vi "setReset.vi"(8 "error":errorcluster, 10 "axis":i32, 11 "connection ID":refnum<k5>) -> (0 "error out":errorcluster, 2 "axis_out":i32, 3 "connection ID out":refnum<k5>)   [LabVIEW 2016, in "amc_api.lvlib"]
doc: "This function resets the actual position of the selected axis given by the NUM sensor to zero and marks the reference position as invalid."
uses:
  amc_api.lvlib
panel:
  out "jsonRespIn":string
  out "JSON-response":string="{\"jsonrpc\":\"2.0\",\"method\":\"\",\"params\":[5,1.245,true,\"name\"],\"id\":\"1\"}"
  out "JSON request":string
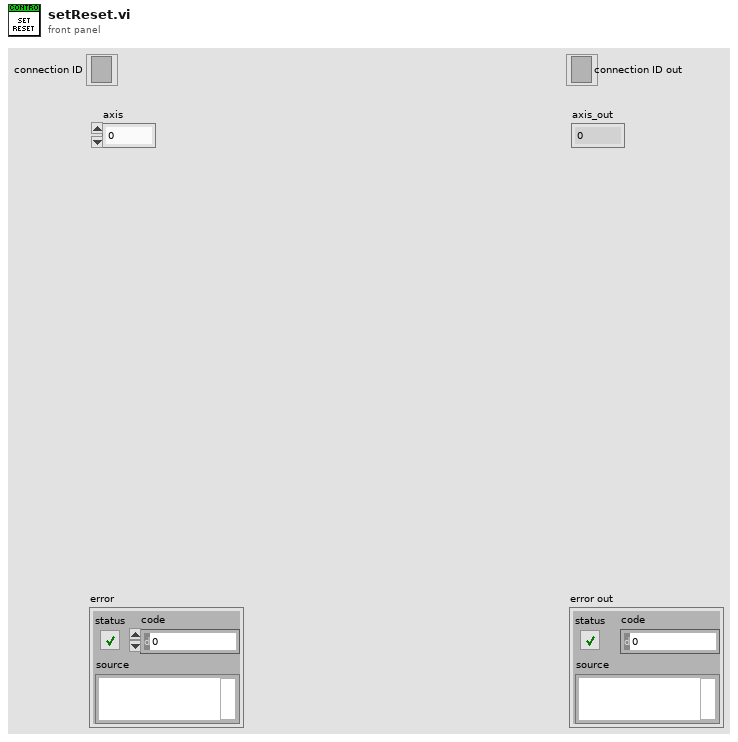
[diagram p1: front panel]
types:
  T1 = cluster{"jsonrpc":string, "method":string, "params":string[], "id":string, "api":i32, "pid":string}
  T2 = enum16{"Standard", "Buffered", "CRLF", "Immediate"}
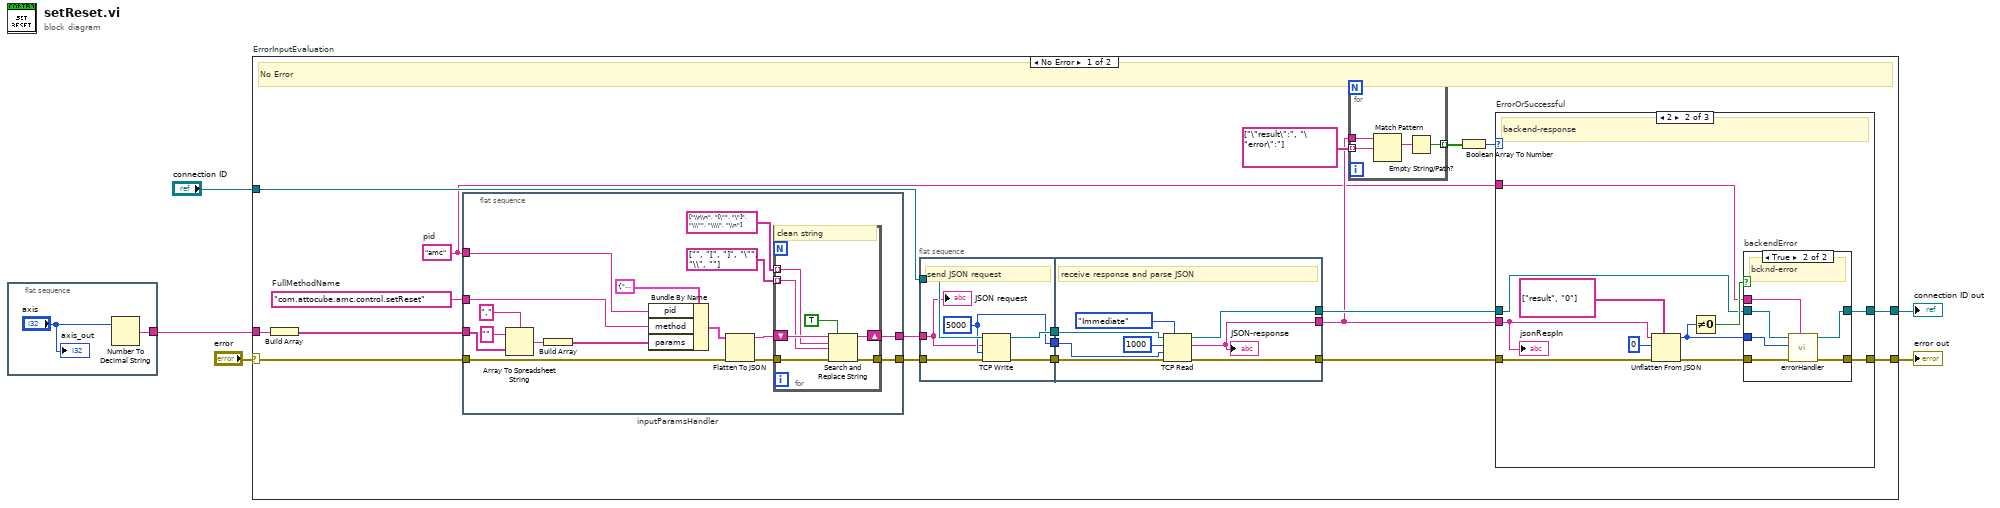
[diagram p0: block diagram]
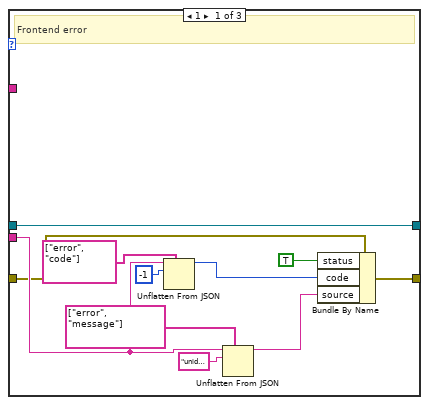
[diagram p2: hidden frame]
diagram:
  n1 = flat-sequence "in_axis" {
    tunnel: [w7] -> w1
    frame #0 {
      n2 = Number To Decimal String(number="axis") -> (decimal integer string=w7:string)  [unwired: 1 in]
      "axis_out" <- "axis"
    }
  }
  n3 = case "ErrorInputEvaluation" shown="No Error" "error" {
    selector: "error" -> [w13 w100]
    tunnel: "connection ID" -> [w23 w101]
    tunnel: [w15 w100] -> w4
    tunnel: [w16 w101] -> w3
    tunnel: w1 -> [w8 _]
    frame No Error {
      w9 = "amc"  # pid
      w14 = "com.attocube.amc.control.setReset"  # FullMethodName
      # "No Error"
      n4 = Build Array ("ParametersArrayString")(w8) -> (w12:string[])
      n5 = flat-sequence "inputParamsHandler" {
        tunnel: [w32] -> w11
        tunnel: w12 -> [w38]
        tunnel: w13 -> [w37]
        tunnel: [w34] -> w10
        tunnel: w14 -> [w28]
        tunnel: w9 -> [w27]
        frame #0 {
          n6 = Array To Spreadsheet String(delimiter (Tab)=",", array=w38, 3:"" ("format string")) -> (spreadsheet string=w40:string)
          n7 = Build Array "Build Array"(w40) -> (w29:string[])
          n8 = Bundle By Name(cluster=T1 {"jsonrpc"="2.0", "method"="com.attocube.amc.res.setRESReadOutFreq", "params"=[], "id"="1", "api"=2, "pid"=""}, "pid"=w27, "method"=w28, "params"=w29) -> (w39:T1)
          n9 = Flatten To JSON(anything=w39, error in (no error)=w37) -> (JSON string=w33:string, 11:w35:errorcluster)  [unwired: 1 in]
          n10 = for {
            tunnel: string[] ["\\r\\n", "[\"", "\"]", "\\\"", "\\\\", "\\n"] ("search string") -> [w46] mode=indexing
            tunnel: string[] ["", "[", "]", "\"", "\\", ""] ("replace string (\"\")") -> [w45] mode=indexing
            shift-right: [w48] -> w32
            shift-left: w33 -> [w47]
            tunnel: w35 -> [w44]
            tunnel: [w43] -> w34
            # "clean string"
            n11 = Search and Replace String(replace all?=TRUE ("replace all? (F)"), input string=w47, search string=w46, replace string=w45, error in=w44) -> (result string=w48:string, error out=w43:errorcluster)  [unwired: 3 in, 2 out]
          }
        }
      }
      n12 = flat-sequence {
        tunnel: w23 -> [w91]
        tunnel: [w89] -> w26
        tunnel: [w90] -> w25
        tunnel: w10 -> [w86]
        tunnel: [w88] -> w24
        tunnel: w11 -> [w87]
        tunnel: [w95] -> w19
        tunnel: w26 -> [w97]
        tunnel: w25 -> [w96]
        tunnel: [w93] -> w18
        tunnel: w24 -> [w94]
        tunnel: [w92] -> w17
        frame #0 {
          w88 = 5000 ("timeout ms (25000)")
          # "send JSON request"
          n13 = TCP Write(connection ID=w91, data in=w87, error in (no error)=w86, 9:w88) -> (connection ID out=w89:refnum<k5>, error out=w90:errorcluster)  [unwired: 1 out]
          "JSON request" <- w87
        }
        frame #1 {
          # "receive response and parse JSON"
          n14 = TCP Read(connection ID=w97, bytes to read=1000, error in (no error)=w96, 7:T2."Immediate" ("mode (standard)"), 9:w94) -> (connection ID out=w95:refnum<k5>, data out=w92:string, error out=w93:errorcluster)
          "JSON-response" <- w92
        }
      }
      n15 = for {
        tunnel: string[] ["\"result\":", "\"error\":"] ("path") -> [w52] mode=indexing
        tunnel: [w50] -> w21 mode=indexing
        tunnel: w17 -> [w53]
        n16 = Match Pattern(string=w53, regular expression=w52) -> (match substring=w51:string)  [unwired: 1 in, 3 out]
        n17 = Empty String/Path?(string/path=w51) -> (empty?=w50:bool)
      }
      n18 = Boolean Array To Number(Boolean array=w21) -> (number=w20:u32)
      n19 = case "ErrorOrSuccessful" shown="2" w20 {
        tunnel: w17 -> [w56 w66 _]
        tunnel: w19 -> [w54 w69 w85]
        tunnel: [w54 w68 w85] -> w16
        tunnel: [w57 w67 w84] -> w15
        tunnel: w18 -> [w55 w70 w84]
        tunnel: w9 -> [_ w65 _]
        frame 1 {
          # "Frontend error"
          n20 = Unflatten From JSON(path=string[] ["error", "code"], JSON string=w56, type and defaults=-1) -> (value=w63:i32)  [unwired: 4 in, 1 out]
          n21 = Unflatten From JSON(path=string[] ["error", "message"], JSON string=w56, type and defaults="unidentified error") -> (value=w64:string)  [unwired: 4 in, 1 out]
          n22 = Bundle By Name(cluster=w55, "status"=TRUE, "code"=w63, "source"=w64) -> (w57:errorcluster)
        }
        frame 2 {
          # "backend-response"
          n23 = Unflatten From JSON(path=string[] ["result", "0"], JSON string=w66, type and defaults=0, error in (no error)=w70) -> (value=w75:i32, error out=w73:errorcluster)  [unwired: 3 in]
          n24 = Not Equal To 0?(x=w75) -> (x != 0?=w74:bool)
          n25 = case "backendError" shown="True" w74 {
            tunnel: w75 -> [_ w83]
            tunnel: w73 -> [w77 w82]
            tunnel: [w76 w81] -> w68
            tunnel: [w77 w80] -> w67
            tunnel: w69 -> [w76 w79]
            tunnel: w65 -> [_ w78]
            frame False {
              # "successful"
            }
            frame True {
              # "bcknd-error"
              n26 = call "errorHandler.vi"("pid"=w78, "error in"=w82, "errNbr"=w83, "connection ID"=w79) -> ("error out 2"=w80:errorcluster, "connection ID out"=w81:refnum<k5>)  [unwired: 6 in]
            }
          }
          "jsonRespIn" <- w66
        }
        frame Default {
          # "NoResponse"
        }
      }
    }
    frame Error {
      # "Error"
    }
  }
  "error out" <- w4
  "connection ID out" <- w3
